vi "1.vi"   [LabVIEW 2023, in "2023.lvlib"]
uses:
  2023.lvlib
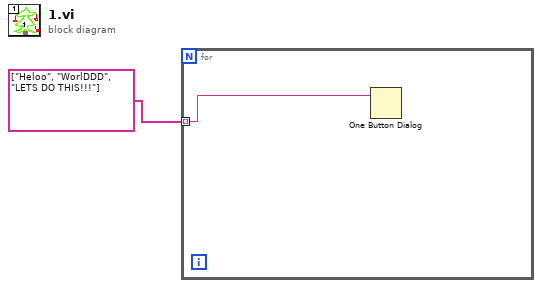
[diagram p0: block diagram]
diagram:
  n1 = for {
    tunnel: string[] ["Heloo", "WorlDDD", "LETS DO THIS!!!"] -> [w2] mode=indexing
    n2 = One Button Dialog(message=w2) -> ()  [unwired: 1 in, 1 out]
  }
